vi "Periodic Tasks.vi"(8 "error in":errorcluster) -> ()   [LabVIEW 2019]
doc: "This VI runs in parallel to other tasks. It can contain as many user-defined periodic loops as you need. These can carry out PID or other sorts of timed response."
uses:
  <vilib>/Rock Robotics/WPI/ThirdParty/Phoenix-LabVIEW/Motor Controller/Controls/CTRE_Phoenix_MotorControl_ControlMode.ctl
  MotorsGlobal.vi
  JoysticksGlobal.vi
  <vilib>/Rock Robotics/WPI/Utilities/WPI_GetSetVariantRefNum.vi
panel:
  in  "PIDs Tab":enum32{"Fly Wheel PID", "Page 2"}(tab)
  in  "EnableFWPID":bool
  out "Variable":dbl
  out "ShooterChart":cluster{"Setpoint":dbl, "Process variable":dbl}(graph)
  in  "FWGains":T1={"proportional gain (Kc)"=1.0, "integral time (Ti, min)"=0.01, "derivative time (Td, min)"=0.0} {"derivative time (Td, min)" format="%.3f"; "integral time (Ti, min)" format="%.3f"; "proportional gain (Kc)" format="%.3f"}
  in  "FWRange":cluster{"output high":dbl, "output low":dbl}={"output high"=0.6, "output low"=-0.6} {"output low" format="%.2f"; "output high" format="%.2f"}
  in  "FWIntegral Range":dbl=10000.0
  in  "FWSetpoint":dbl
  in  "FWDisable Range":dbl
  in  "EnableTest":bool
  in  "MotorInput":dbl=0.6
  # "System Tester"
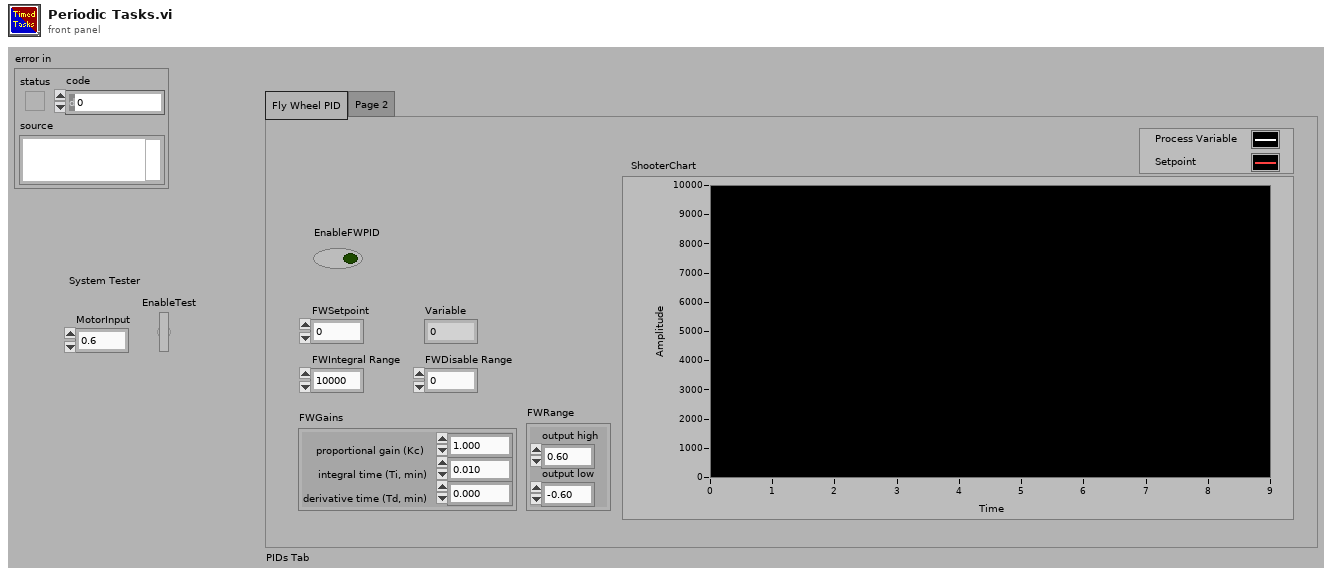
[diagram p1: front panel]
types:
  T1 = cluster{"proportional gain (Kc)":dbl, "integral time (Ti, min)":dbl, "derivative time (Td, min)":dbl}
  T2 = typedef "WPI_MotorControlDeviceRef.ctl" = cluster{"DeviceStatus":errorcluster, "Type":T3, "PWM":cluster{"PWM Channel":T4, "DeadBand":T5}, "CAN":cluster{"Device Number":u8, "SetOutput VI Ref":variant, "GetOutput VI Ref":variant, "Enable VI Ref":variant, "Disable VI Ref":variant, "Data":variant}, "Invert":bool, "DIO PWM":cluster{"PWM \"Enable\" Channel":T4, "DIOChannel":T6, "PWM Rate":dbl}}
  T3 = typedef "WPI_MotorControlType.ctl" = enum16{"PWM", "CAN", "DIO PWM"}
  T4 = typedef "FPGA_DIOPWMChannel.ctl" = enum8{"PWM 0", "PWM 1", "PWM 2", "PWM 3", "PWM 4", "PWM 5", "PWM 6", "PWM 7", "PWM 8", "PWM 9", "PWM MXP 0", "PWM MXP 1", "PWM MXP 2", "PWM MXP 3", "PWM MXP 4", "PWM MXP 5", "PWM MXP 6", "PWM MXP 7", "PWM MXP 8", "PWM MXP 9", "Invalid"}
  T5 = typedef "WPI_PWMDeadband.ctl" = cluster{"Name":string, "maxPositivePwm":i32, "minPositivePwm":i32, "centerPwm":i32, "maxNegativePwm":i32, "minNegativePwm":i32, "angularRange":u16}
  T6 = typedef "FPGA_DIOChannel.ctl" = enum8{"DIO 0", "DIO 1", "DIO 2", "DIO 3", "DIO 4", "DIO 5", "DIO 6", "DIO 7", "DIO 8", "DIO 9", "DIO MXP 0", "DIO MXP 1", "DIO MXP 2", "DIO MXP 3", "DIO MXP 4", "DIO MXP 5", "DIO MXP 6", "DIO MXP 7", "DIO MXP 8", "DIO MXP 9", "DIO MXP 10", "DIO MXP 11", "DIO MXP 12", "DIO MXP 13", "DIO MXP 14", "DIO MXP 15", "SPI Port CS1", "SPI Port CS2", "SPI Port CS3", "SPI Port MISO", "SPI Port MOSI", "Invalid"}
  T7 = typedef "WPI_EncoderDevRef.ctl" = cluster{"DevStatus":errorcluster, "EncoderIndex":T8, "CounterIndex":T9, "DistancePerCount":dbl, "Decoding Type":T10}
  T8 = typedef "FPGA_EncoderIdx.ctl" = enum8{"Enc 0", "Enc 1", "Enc 2", "Enc 3", "Enc 4", "Enc 5", "Enc 6", "Enc 7", "Invalid"}
  T9 = typedef "FPGA_CounterCtrSystemIndex.ctl" = enum8{"Ctr 0", "Ctr 1", "Ctr 2", "Ctr 3", "Ctr 4", "Ctr 5", "Ctr 6", "Ctr 7", "Invalid"}
  T10 = typedef "WPI_EncoderType.ctl" = enum16{"1x", "2x", "4x"}
  T11 = typedef "CTRE_Phoenix_MotorControl_ControlMode.ctl" = u16
  T12 = typedef "WPI_RobotDriveDevRef.ctl" = cluster{"DevStatus":errorcluster, "Motors[]":T2[], "Square Inputs":bool, "Max Output":dbl}
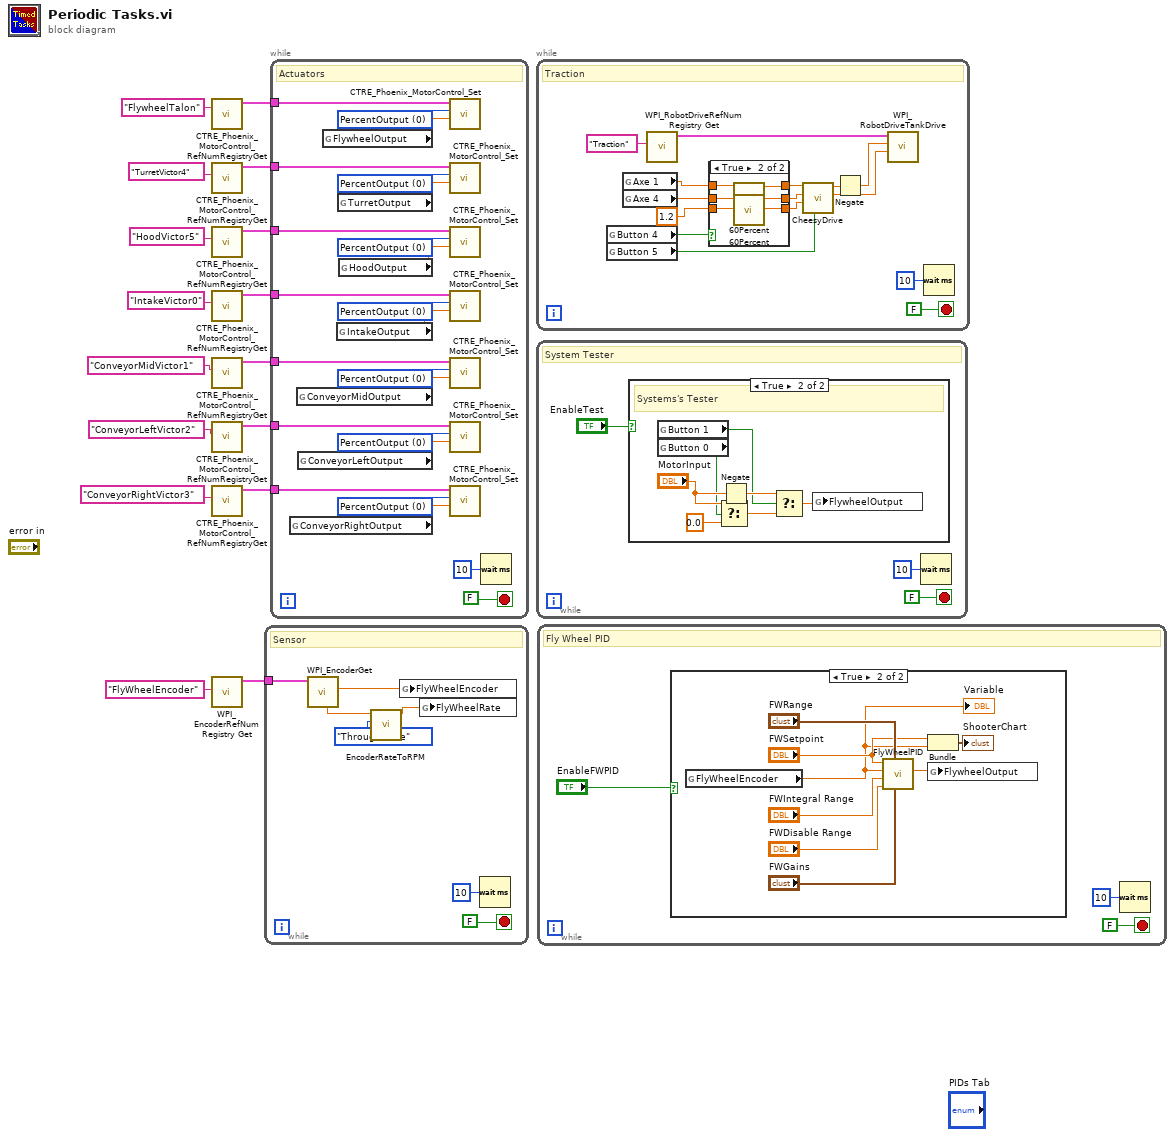
[diagram p0: block diagram]
diagram:
  n1 = call <vilib>:"CTRE_Phoenix_MotorControl_RefNumRegistryGet.vi"("refnum name"="FlywheelTalon") -> ("PhoenixMotorControlDevRef"=w15:T2)  [unwired: 9 in, 1 out]
  n2 = call <vilib>:"CTRE_Phoenix_MotorControl_RefNumRegistryGet.vi"("refnum name"="TurretVictor4") -> ("PhoenixMotorControlDevRef"=w13:T2)  [unwired: 9 in, 1 out]
  n3 = call <vilib>:"CTRE_Phoenix_MotorControl_RefNumRegistryGet.vi"("refnum name"="HoodVictor5") -> ("PhoenixMotorControlDevRef"=w14:T2)  [unwired: 9 in, 1 out]
  n4 = call <vilib>:"CTRE_Phoenix_MotorControl_RefNumRegistryGet.vi"("refnum name"="IntakeVictor0") -> ("PhoenixMotorControlDevRef"=w10:T2)  [unwired: 9 in, 1 out]
  n5 = call <vilib>:"CTRE_Phoenix_MotorControl_RefNumRegistryGet.vi"("refnum name"="ConveyorMidVictor1") -> ("PhoenixMotorControlDevRef"=w9:T2)  [unwired: 9 in, 1 out]
  n6 = call <vilib>:"CTRE_Phoenix_MotorControl_RefNumRegistryGet.vi"("refnum name"="ConveyorLeftVictor2") -> ("PhoenixMotorControlDevRef"=w8:T2)  [unwired: 9 in, 1 out]
  n7 = call <vilib>:"CTRE_Phoenix_MotorControl_RefNumRegistryGet.vi"("refnum name"="ConveyorRightVictor3") -> ("PhoenixMotorControlDevRef"=w7:T2)  [unwired: 9 in, 1 out]
  n8 = call <vilib>:"WPI_EncoderRefNum Registry Get.vi"("refnum name"="FlyWheelEncoder") -> ("EncoderDevRef"=w2:T7)  [unwired: 9 in, 1 out]
  n9 = while {
    tunnel: w2 -> [w21]
    stop <- FALSE stop-if-true
    # "Sensor"
    n10 = call <vilib>:"WPI_EncoderGet.vi"("EncoderDevRef"=w21) -> ("Distance"=w20:dbl, "Rate"=w19:dbl)  [unwired: 5 in, 4 out]
    n11 = call "EncoderRateToRPM.vi"("Enum"=enum16{"Through Bore", "Mag"}."Through Bore", "EncoderRate"=w19) -> ("RPS"=w18:dbl)  [unwired: 8 in, 1 out]
    n12 = global write "MotorsGlobal.vi" "FlyWheelEncoder"(w20) -> ()
    n13 = global write "MotorsGlobal.vi" "FlyWheelRate"(w18) -> ()
    n14 = Wait (ms)(milliseconds to wait=u32 10) -> ()  [unwired: 1 out]
  }
  n15 = while {
    tunnel: w15 -> [w43]
    tunnel: w14 -> [w42]
    tunnel: w13 -> [w41]
    tunnel: w10 -> [w35]
    tunnel: w9 -> [w34]
    tunnel: w8 -> [w33]
    tunnel: w7 -> [w32]
    stop <- FALSE stop-if-true
    w25 = T11 0 items=["PercentOutput"=0, "Position"=1, "Velocity"=2, "Current"=3, "Follower"=5, "MotionProfile"=6, "MotionMagic"=7, "MotionProfileArc"=10, "Disabled"=15] ("Control Mode")
    w27 = T11 0 items=["PercentOutput"=0, "Position"=1, "Velocity"=2, "Current"=3, "Follower"=5, "MotionProfile"=6, "MotionMagic"=7, "MotionProfileArc"=10, "Disabled"=15] ("Control Mode")
    w29 = T11 0 items=["PercentOutput"=0, "Position"=1, "Velocity"=2, "Current"=3, "Follower"=5, "MotionProfile"=6, "MotionMagic"=7, "MotionProfileArc"=10, "Disabled"=15] ("Control Mode")
    w31 = T11 0 items=["PercentOutput"=0, "Position"=1, "Velocity"=2, "Current"=3, "Follower"=5, "MotionProfile"=6, "MotionMagic"=7, "MotionProfileArc"=10, "Disabled"=15] ("Control Mode")
    w39 = T11 0 items=["PercentOutput"=0, "Position"=1, "Velocity"=2, "Current"=3, "Follower"=5, "MotionProfile"=6, "MotionMagic"=7, "MotionProfileArc"=10, "Disabled"=15] ("Control Mode")
    w38 = T11 0 items=["PercentOutput"=0, "Position"=1, "Velocity"=2, "Current"=3, "Follower"=5, "MotionProfile"=6, "MotionMagic"=7, "MotionProfileArc"=10, "Disabled"=15] ("Control Mode")
    w44 = T11 0 items=["PercentOutput"=0, "Position"=1, "Velocity"=2, "Current"=3, "Follower"=5, "MotionProfile"=6, "MotionMagic"=7, "MotionProfileArc"=10, "Disabled"=15] ("Control Mode")
    # "Actuators"
    n16 = global read "MotorsGlobal.vi" "ConveyorRightOutput"() -> (w24:dbl)
    n17 = global read "MotorsGlobal.vi" "ConveyorMidOutput"() -> (w28:dbl)
    n18 = global read "MotorsGlobal.vi" "ConveyorLeftOutput"() -> (w26:dbl)
    n19 = global read "MotorsGlobal.vi" "FlywheelOutput"() -> (w40:dbl)
    n20 = global read "MotorsGlobal.vi" "IntakeOutput"() -> (w30:dbl)
    n21 = global read "MotorsGlobal.vi" "TurretOutput"() -> (w37:dbl)
    n22 = global read "MotorsGlobal.vi" "HoodOutput"() -> (w36:dbl)
    n23 = call <vilib>:"CTRE_Phoenix_MotorControl_Set.vi"("Output"=w40, "Control Mode"=w44, "PhoenixMotorControlDevRef"=w43) -> ()  [unwired: 7 in, 2 out]
    n24 = call <vilib>:"CTRE_Phoenix_MotorControl_Set.vi"("Output"=w37, "Control Mode"=w38, "PhoenixMotorControlDevRef"=w41) -> ()  [unwired: 7 in, 2 out]
    n25 = call <vilib>:"CTRE_Phoenix_MotorControl_Set.vi"("Output"=w36, "Control Mode"=w39, "PhoenixMotorControlDevRef"=w42) -> ()  [unwired: 7 in, 2 out]
    n26 = call <vilib>:"CTRE_Phoenix_MotorControl_Set.vi"("Output"=w30, "Control Mode"=w31, "PhoenixMotorControlDevRef"=w35) -> ()  [unwired: 7 in, 2 out]
    n27 = call <vilib>:"CTRE_Phoenix_MotorControl_Set.vi"("Output"=w28, "Control Mode"=w29, "PhoenixMotorControlDevRef"=w34) -> ()  [unwired: 7 in, 2 out]
    n28 = call <vilib>:"CTRE_Phoenix_MotorControl_Set.vi"("Output"=w26, "Control Mode"=w27, "PhoenixMotorControlDevRef"=w33) -> ()  [unwired: 7 in, 2 out]
    n29 = call <vilib>:"CTRE_Phoenix_MotorControl_Set.vi"("Output"=w24, "Control Mode"=w25, "PhoenixMotorControlDevRef"=w32) -> ()  [unwired: 7 in, 2 out]
    n30 = Wait (ms)(milliseconds to wait=u32 10) -> ()  [unwired: 1 out]
  }
  n31 = while {
    stop <- FALSE stop-if-true
    # "Traction"
    n32 = global read "JoysticksGlobal.vi" "Button 4"() -> (w53:bool)
    n33 = global read "JoysticksGlobal.vi" "Button 5"() -> (w54:bool)
    n34 = global read "JoysticksGlobal.vi" "Axe 1"() -> (w50:dbl)
    n35 = global read "JoysticksGlobal.vi" "Axe 4"() -> (w52:dbl)
    n36 = call <vilib>:"WPI_RobotDriveRefNum Registry Get.vi"("refnum name"="Traction") -> ("RobotDriveDevRef"=w59:T12)  [unwired: 9 in, 1 out]
    n37 = case shown="True" w53 {
      tunnel: [w64 w68] -> w51
      tunnel: w52 -> [w64 w69]
      tunnel: [w63 w67] -> w49
      tunnel: w50 -> [w63 w66]
      tunnel: 1.2 ("Sensitivty") -> [w62 w65]
      tunnel: [w62 w65] -> w47
      frame False {
      }
      frame True {
        n38 = call "60Percent.vi"("In"=w66) -> ("Out"=w67:dbl)  [unwired: 9 in]
        n39 = call "60Percent.vi"("In"=w69) -> ("Out"=w68:dbl)  [unwired: 9 in]
      }
    }
    n40 = call "CheesyDrive.vi"("Quickturn"=w54, "Sensitivty"=w47, "Wheel"=w51, "Throttle"=w49) -> ("Right PWM"=w56:dbl, "Left PWM"=w57:dbl)  [unwired: 6 in]
    n41 = Negate(x=w57) -> (-x=w55:dbl)
    n42 = call <vilib>:"WPI_RobotDriveTankDrive.vi"("Right axis value"=w56, "Left axis value"=w55, "RobotDriveDevRef"=w59) -> ()  [unwired: 6 in, 3 out]
    n43 = Wait (ms)(milliseconds to wait=u32 10) -> ()  [unwired: 1 out]
  }
  n44 = while {
    stop <- FALSE stop-if-true
    # "System Tester"
    n45 = case shown="True" "EnableTest" {
      frame False {
      }
      frame True {
        # "Systems's Tester"
        n46 = global read "JoysticksGlobal.vi" "Button 1"() -> (w75:bool)
        n47 = global read "JoysticksGlobal.vi" "Button 0"() -> (w76:bool)
        n48 = Select(t="MotorInput", s=w76, f=0.0) -> (s? t:f=w79:dbl)
        n49 = Negate(x="MotorInput") -> (-x=w77:dbl)
        n50 = Select(t=w77, s=w75, f=w79) -> (s? t:f=w73:dbl)
        n51 = global write "MotorsGlobal.vi" "FlywheelOutput"(w73) -> ()
      }
    }
    n52 = Wait (ms)(milliseconds to wait=u32 10) -> ()  [unwired: 1 out]
  }
  n53 = while {
    stop <- FALSE stop-if-true
    # "Fly Wheel PID"
    n54 = case shown="True" "EnableFWPID" {
      frame False {
      }
      frame True {
        n55 = global read "MotorsGlobal.vi" "FlyWheelEncoder"() -> (w83:dbl)
        "Variable" <- w83
        n56 = call "FlyWheelPID.vi"("FWGains"="FWGains", "FWRange"="FWRange", "FWDisable Range"="FWDisable Range", "FWIntegral Range"="FWIntegral Range", "FWProcess variable"=w83, "FWSetpoint"="FWSetpoint") -> ("FWoutput"=w86:dbl)  [unwired: 4 in]
        n57 = Bundle("FWSetpoint"="FWSetpoint", "FlyWheelEncoder"=w83) -> (→"ShooterChart":cluster{"FWSetpoint":dbl, "FlyWheelEncoder":dbl})  [unwired: 1 in]
        n58 = global write "MotorsGlobal.vi" "FlywheelOutput"(w86) -> ()
      }
    }
    n59 = Wait (ms)(milliseconds to wait=u32 10) -> ()  [unwired: 1 out]
  }
